vi "Build Links Application.vi"(8 "error in":errorcluster) -> (0 "error out":errorcluster, 3 "Path to Application":path)   [LabVIEW 2014]
uses:
  <vilib>/AppBuilder/AB_API_Simple/Build (path).vi
  <vilib>/AppBuilder/AB_API_Simple/NI_App_Builder_API.lvlib
panel:
  # "Inputs"
  # "Outputs"
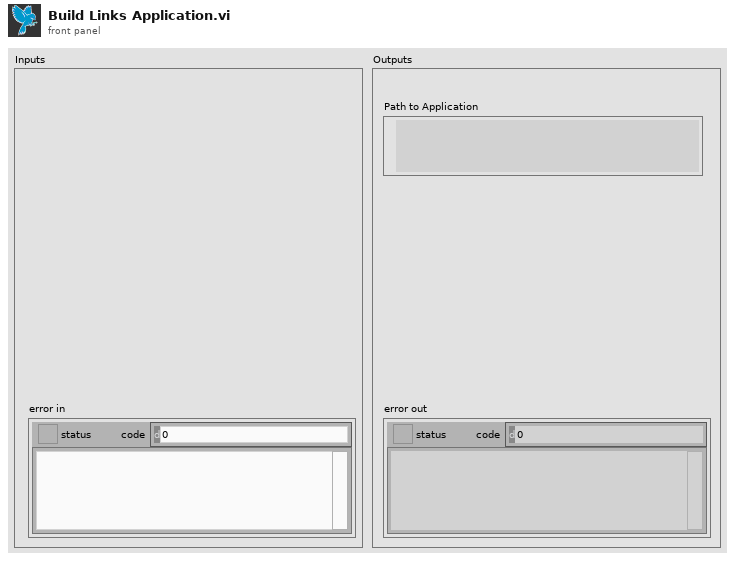
[diagram p1: front panel]
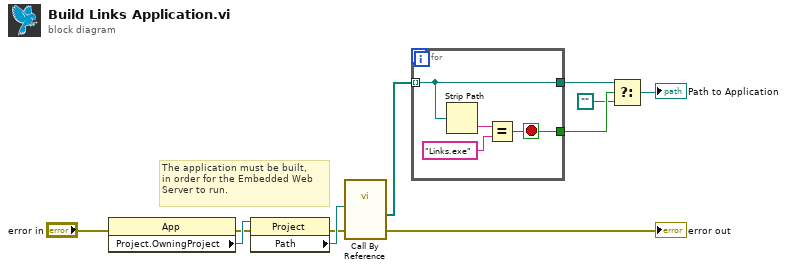
[diagram p0: block diagram]
diagram:
  # "The application must be built,\nin order for the Embedded Web\nServer to run."
  n1 = property class="App"(error in="error in") -> (error out=w9:errorcluster, "Project.OwningProject"=w10:refnum<vi>)  [unwired: 1 in, 1 out]
  n2 = property class="Project"(reference=w10, error in=w9) -> (error out=w7:errorcluster, "Path"=w8:path)  [unwired: 1 out]
  n3 = call-by-ref "?"("error in (no error)"=w7, "Path to project"=w8) -> ("error out"=→"error out":errorcluster, "Generated files"=w11:path[])  [unwired: 10 in, 2 out]
  n4 = for {
    tunnel: w11 -> [w12] mode=indexing
    tunnel: [w12] -> w3
    tunnel: [w13] -> w4
    stop <- w13 stop-if-true
    n5 = Strip Path(path=w12) -> (name=w15:string)  [unwired: 1 out]
    n6 = Equal?(x=w15, y="Links.exe") -> (x = y?=w13:bool)
  }
  n7 = Select(t=w3, s=w4, f=path "") -> (s? t:f=→"Path to Application":path)
